vi "Prevent_Overload.vi"(8 "error in":errorcluster, 10 "Channel":i32(ring)=1 items=["Channel 1"=1, "Channel 2"=2, "Channel 3"=3, "Channel 4"=4, "Function 1"=5, "Function 2"=6, "Function 3"=7, "Function 4"=8, "Memory 1"=9, "Memory 2"=10, "Memory 3"=11, "Memory 4"=12], 11 "VISA resource name":refnum<visa-resource-name>) -> (0 "error out":errorcluster, 3 "VISA resource name out":refnum<visa-resource-name>)   [LabVIEW 2009]
uses:
  <instrlib>/Agilent 8000 Series/Agilent 8000 Series.lvlib
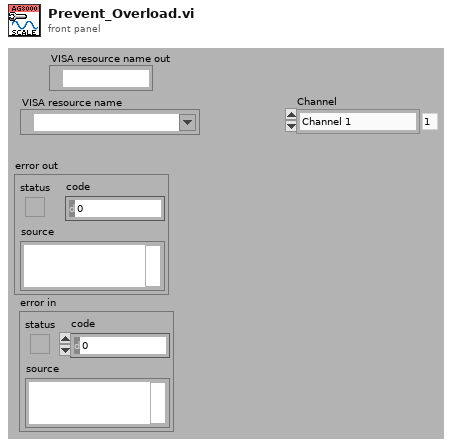
[diagram p1: front panel]
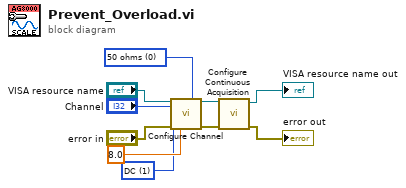
[diagram p0: block diagram]
diagram:
  w1 = 1 items=["AC", "DC"] ("Vertical Coupling (1: DC)")
  w10 = u32 0 items=["50 ohms", "1 Mohms"] ("Input Impedance (1: 1 Mohms)")
  n1 = call <instrlib>:"Configure Channel.vi"("VISA resource name"="VISA resource name", "Input Impedance (1: 1 Mohms)"=w10, "Channel (1: Channel 1)"="Channel", "Vertical Coupling (1: DC)"=w1, "error in (no error)"="error in", "Vertical Range (2.0 V)"=8.0) -> ("VISA resource name out"=w9:refnum<visa-resource-name>, "error out"=w8:errorcluster)  [unwired: 8 in]
  n2 = call <instrlib>:"Configure Continuous Acquisition.vi"("error in (no error)"=w8, "VISA resource name"=w9) -> ("error out"=→"error out":errorcluster, "VISA resource name out"=→"VISA resource name out":refnum<visa-resource-name>)  [unwired: 8 in]
